vi "negate meas mag.vi"(10 "current phi (deg)":dbl, 11 "target phi (deg)":dbl) -> (4 "Negate measured mag?":bool)   [LabVIEW 2013]
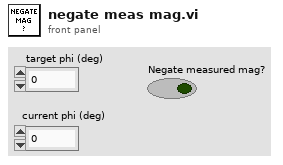
[diagram p1: front panel]
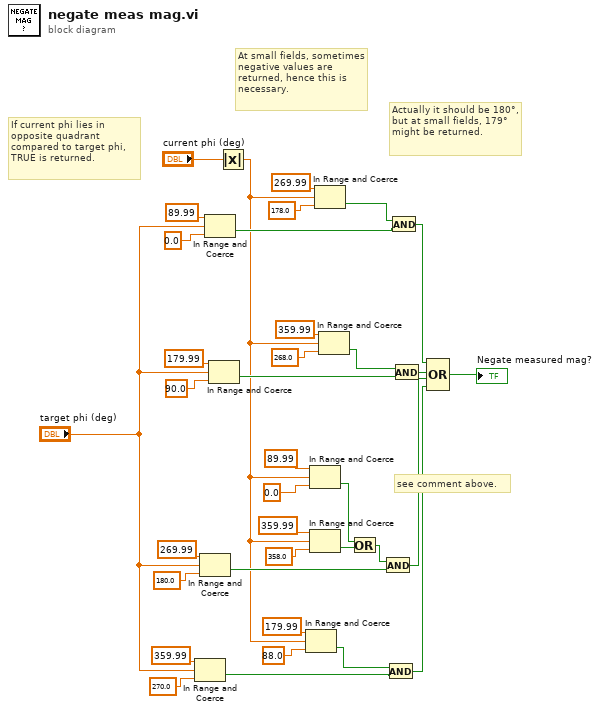
[diagram p0: block diagram]
diagram:
  # "see comment above."
  # "At small fields, sometimes negative values are returned, hence this is necessary."
  # "Actually it should be 180°, but at small fields, 179° might be returned."
  # "If current phi lies in opposite quadrant compared to target phi, TRUE is returned."
  n1 = In Range and Coerce(upper limit=359.99, x="target phi (deg)", lower limit=270.0) -> (In Range?=w21:bool)  [unwired: 1 out]
  n2 = In Range and Coerce(upper limit=269.99, x="target phi (deg)", lower limit=180.0) -> (In Range?=w34:bool)  [unwired: 1 out]
  n3 = In Range and Coerce(upper limit=89.99, x="target phi (deg)", lower limit=0.0) -> (In Range?=w26:bool)  [unwired: 1 out]
  n4 = In Range and Coerce(upper limit=179.99, x="target phi (deg)", lower limit=90.0) -> (In Range?=w13:bool)  [unwired: 1 out]
  n5 = Absolute Value(x="current phi (deg)") -> (abs(x)=w1:dbl)
  n6 = In Range and Coerce(upper limit=179.99, x=w1, lower limit=88.0) -> (In Range?=w20:bool)  [unwired: 1 out]
  n7 = In Range and Coerce(upper limit=89.99, x=w1, lower limit=0.0) -> (In Range?=w5:bool)  [unwired: 1 out]
  n8 = In Range and Coerce(upper limit=359.99, x=w1, lower limit=358.0) -> (In Range?=w2:bool)  [unwired: 1 out]
  n9 = In Range and Coerce(upper limit=269.99, x=w1, lower limit=178.0) -> (In Range?=w27:bool)  [unwired: 1 out]
  n10 = In Range and Coerce(upper limit=359.99, x=w1, lower limit=268.0) -> (In Range?=w12:bool)  [unwired: 1 out]
  n11 = Or(x=w5, y=w2) -> (x .or. y?=w6:bool)
  n12 = And(x=w6, y=w34) -> (x .and. y?=w36:bool)
  n13 = And(x=w20, y=w21) -> (x .and. y?=w29:bool)
  n14 = And(x=w27, y=w26) -> (x .and. y?=w28:bool)
  n15 = And(x=w12, y=w13) -> (x .and. y?=w14:bool)
  n16 = Compound Arithmetic op=OR(w28, w14, w36, w29) -> (→"Negate measured mag?":bool)
